vi "regex test.vi"() -> ()   [LabVIEW 2016, in "labssh_thijs.lvlib"]
uses:
  <vilib>/regexp/Match Regular Expression.xnode
  labssh_thijs.lvlib
panel:
  out "prompt before $ sign":string
  out "after match 3":string
  out "whole match 3":string
  out "before match 2":string
  out "final match":string
  out "after match 2":string
  out "whole match 2":string
  out "prompt and space":string
  out "after match":string
  out "whole match":string
  out "before match":string
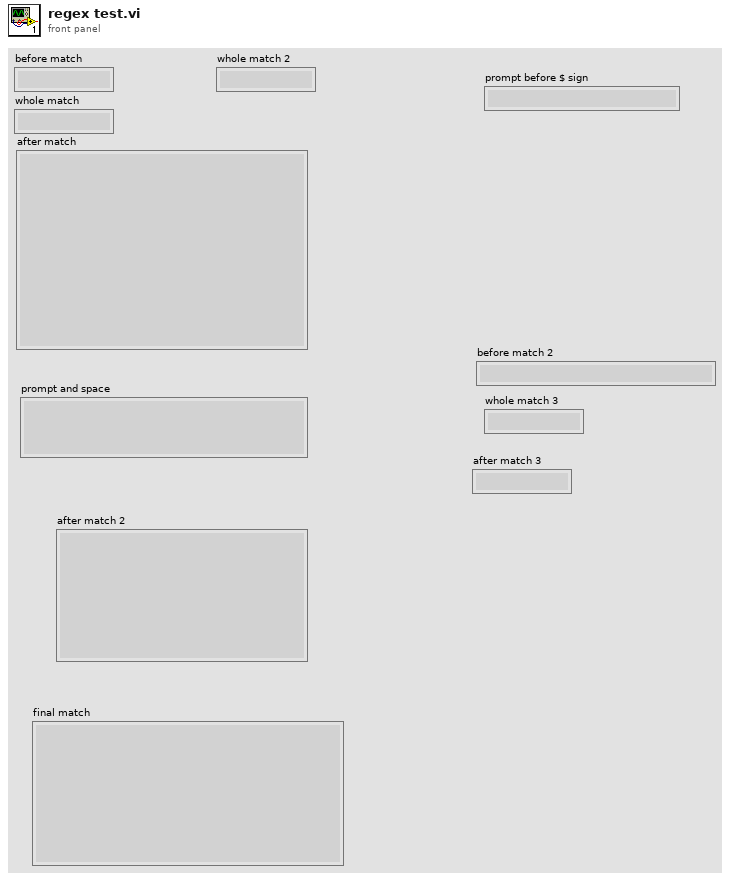
[diagram p1: front panel]
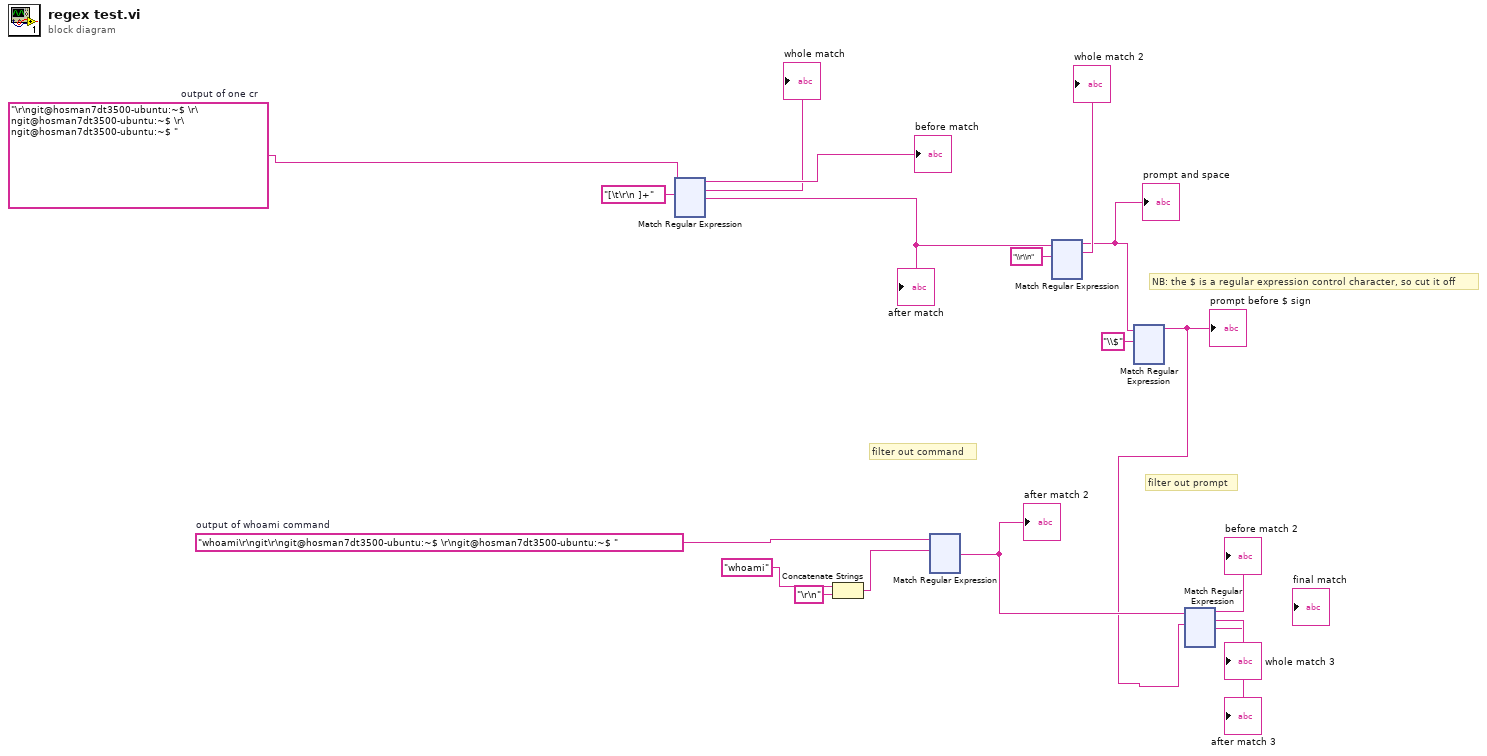
[diagram p0: block diagram]
diagram:
  w11 = "whoami\r\ngit\r\ngit@hosman7dt3500-ubuntu:~$ \r\ngit@hosman7dt3500-ubuntu:~$ "  # output of whoami command
  w15 = "\r\ngit@hosman7dt3500-ubuntu:~$ \r\ngit@hosman7dt3500-ubuntu:~$ \r\ngit@hosman7dt3500-ubuntu:~$ "  # output of one cr
  # "NB: the $ is a regular expression control character, so cut it off"
  # "filter out prompt"
  # "filter out command"
  n1 = xnode "Match Regular Expression"("input string"=w15, "regular expression"="[\t\r\n ]+") -> ("before match"=→"before match":string, "whole match"=→"whole match":string, "after match"=w14:string)  [unwired: 4 in, 2 out]
  "after match" <- w14
  n2 = Concatenate Strings("whoami" ("regular expression"), "\r\n" ("string")) -> (w8:string)
  n3 = xnode "Match Regular Expression"("input string"=w11, "regular expression"=w8) -> ("after match"=w7:string)  [unwired: 4 in, 4 out]
  "after match 2" <- w7
  n4 = xnode "Match Regular Expression"("input string"=w14, "regular expression"="\\r\\n") -> ("before match"=w3:string, "whole match"=→"whole match 2":string)  [unwired: 4 in, 3 out]
  "prompt and space" <- w3
  n5 = xnode "Match Regular Expression"("input string"=w3, "regular expression"="\\$") -> ("before match"=w1:string)  [unwired: 4 in, 4 out]
  "prompt before $ sign" <- w1
  n6 = xnode "Match Regular Expression"("input string"=w7, "regular expression"=w1) -> ("before match"=→"before match 2":string, "whole match"=→"whole match 3":string, "after match"=→"after match 3":string)  [unwired: 4 in, 2 out]
